vi "Integer To ASCII Code.vi"(10 "Numeric In":u8) -> (2 "ASCII Code Out":string)   [LabVIEW 2024]
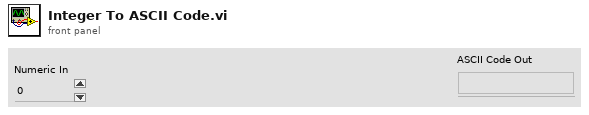
[diagram p1: front panel]
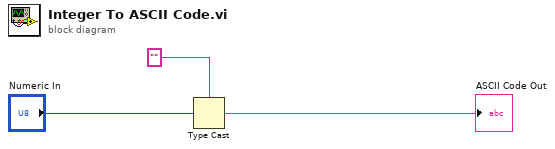
[diagram p0: block diagram]
diagram:
  n1 = Type Cast(type="", x="Numeric In") -> (*(type *) &x=→"ASCII Code Out":string)
